vi "Global_CMD to SM Data.vi"() -> ()   [LabVIEW 2017, in "WCDrive2018.lvlib"]
uses:
  WCDrive2018.lvlib
  Cluster_CMD to SM Data.ctl
  Enum_SM Cmd Select.ctl
panel:
  in  "CMD Drive Data 2":T1
  in  "CMD Drive Data":T1
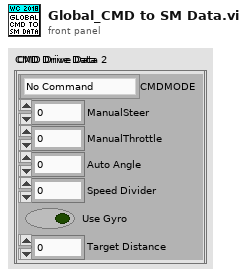
[diagram p1: front panel]
types:
  T1 = typedef "WCDrive2018.lvlib/Cluster_CMD to SM Data.ctl" = cluster{"CMDMODE":T2, "ManualSteer":dbl, "ManualThrottle":dbl, "Auto Angle":dbl, "Speed Divider":dbl, "Use Gyro":bool, "Target Distance":dbl}
  T2 = typedef "WCDrive2018.lvlib/Enum_SM Cmd Select.ctl" = enum16{"No Command", "Halt", "Manual Keep Rotation", "Manual", "Track Front", "Track Rotation"}
diagram:
